vi "conditioning_behavior_120720.vi"() -> ()   [LabVIEW 2019]
doc: "The myRIO Project template acquires acceleration data from the onboard accelerometer and displays the changes of acceleration values in a waveform chart."
uses:
  <vilib>/myRIO/Common/Instrument Driver Framework/myRIO v1.0/Encoder/typedefs/Encoder Signal Mode.ctl
  <vilib>/myRIO/Instrument Drivers/Onboard IO/Encoder/typedefs/Encoder Reference.ctl
  <vilib>/myRIO/Common/Instrument Driver Framework/Utilities/typedefs/myRIO Generic Hardware Reference.ctl
  <vilib>/myRIO/Common/Instrument Driver Framework/Utilities/typedefs/Hardware Version Enum.ctl
  <vilib>/myRIO/Common/Instrument Driver Framework/Utilities/typedefs/myRIO v1.0 Reference.ctl
  <vilib>/myRIO/Common/Instrument Driver Framework/Utilities/typedefs/Generic FPGA Reference.ctl
  <vilib>/myRIO/Common/Instrument Driver Framework/myRIO v1.0/Encoder/typedefs/Encoder Channels Enum.ctl
  <vilib>/myRIO/Common/Instrument Driver Framework/myRIO v1.0/Encoder/typedefs/Encoder Configuration v1.0.ctl
  <vilib>/userdefined/High Color/nirio_resource_hc.ctl
  <vilib>/myRIO/Instrument Drivers/Onboard IO/DIO/typedefs/DIO Reference.ctl
  <vilib>/myRIO/Common/Instrument Driver Framework/myRIO v1.0/DIO/typedefs/DIO Channels List.ctl
  <vilib>/myRIO/Common/Instrument Driver Framework/myRIO v1.0/DIO/typedefs/DIO Channels Enum.ctl
  <vilib>/myRIO/Common/Instrument Driver Framework/Utilities/vis/Is FPGA Ref Available.vi
  <vilib>/myRIO/Common/Instrument Driver Framework/myRIO v1.0/Encoder/vis/myRIO v1.1 Open Encoder.vi
  <vilib>/myRIO/Instrument Drivers/Onboard IO/Encoder/vis/Read.vi
  <vilib>/myRIO/Common/Instrument Driver Framework/myRIO v1.0/DIO/vis/myRIO v1.1 Open DIO.vi
  <vilib>/myRIO/Instrument Drivers/Onboard IO/DIO/vis/Write.vi
  <vilib>/myRIO/Instrument Drivers/Onboard IO/DIO/vis/Read.vi
  <vilib>/myRIO/Common/Instrument Driver Framework/Utilities/vis/Validate Channels.vi
  <vilib>/myRIO/Common/Instrument Driver Framework/myRIO v1.0/Encoder/vis/myRIO v1.0 Reserve Encoder.vi
  <vilib>/myRIO/Common/Instrument Driver Framework/myRIO v1.0/DIO/vis/myRIO v1.0 Reserve DIO.vi
  <vilib>/myRIO/Common/Instrument Driver Framework/myRIO v1.0/Encoder/vis/myRIO v1.0 Build MUX Configuration Encoder.vi
  <vilib>/myRIO/Common/Instrument Driver Framework/myRIO v1.0/Resource Manager/vis/myRIO v1.0 Reserve Channel List.vi
  <vilib>/myRIO/Common/Instrument Driver Framework/myRIO v1.0/DIO/vis/myRIO v1.0 Build MUX Configuration DIO.vi
  <vilib>/myRIO/Common/Instrument Driver Framework/myRIO v1.0/Resource Manager/vis/myRIO v1.0 Create Configuration List.vi
  <vilib>/myRIO/Common/Instrument Driver Framework/myRIO v1.0/Resource Manager/vis/myRIO v1.0 Reserve Channel.vi
  <vilib>/myRIO/Common/Instrument Driver Framework/myRIO v1.0/Resource Manager/vis/myRIO v1.0 Unreserve Channel.vi
  <vilib>/myRIO/Common/Instrument Driver Framework/myRIO v1.0/Resource Manager/vis/myRIO v1.0 Build Mutex Name.vi
  <vilib>/Utility/VariantDataType/GetNumericInfo.vi
  <vilib>/Utility/error.llb/Error Cluster From Error Code.vi
  <vilib>/myRIO/Common/Instrument Driver Framework/myRIO v1.0/myRIO v1.1 Open.vi
  <vilib>/myRIO/Common/Instrument Driver Framework/Utilities/vis/IO Manager.vi
  <vilib>/myRIO/Common/Instrument Driver Framework/Utilities/vis/Configuration Manager.vi
  <vilib>/myRIO/Common/Instrument Driver Framework/myRIO v1.0/Resource Manager/vis/myRIO v1.0 Configure IO.vi
  <vilib>/myRIO/Common/Instrument Driver Framework/myRIO v1.0/myRIO v1.0 Close.vi
  <vilib>/myRIO/Common/Instrument Driver Framework/myRIO v1.0/Encoder/vis/myRIO v1.0 Configure Encoder.vi
  <vilib>/myRIO/Common/Instrument Driver Framework/myRIO v1.0/Encoder/vis/myRIO v1.0 Read Encoder.vi
  <vilib>/myRIO/Common/Instrument Driver Framework/myRIO v1.0/DIO/vis/myRIO v1.0 Read DIO.vi
  <vilib>/myRIO/Common/Instrument Driver Framework/myRIO v1.0/DIO/vis/myRIO v1.0 Write DIO.vi
  <vilib>/myRIO/Express VI/Onboard IO/Encoder/Encoder Express VI.xnode
  <vilib>/myRIO/Instrument Drivers/Onboard IO/Encoder/vis/myRIO Encoder Open.xnode
  <vilib>/myRIO/Express VI/Onboard IO/DI/DI Express VI.xnode
  <vilib>/myRIO/Instrument Drivers/Onboard IO/DIO/vis/myRIO DIO Open.xnode
  <vilib>/myRIO/Express VI/Onboard IO/DO/DO Express VI.xnode
  <vilib>/myRIO/Instrument Drivers/Onboard IO/Encoder/Encoder.lvlib
  <vilib>/myRIO/Instrument Drivers/Onboard IO/DIO/DIO.lvlib
panel:
  out "Frame clock":i32
  out "Reward":bool=TRUE
  in  "Give reward":bool
  out "Licks":u32
  out "Lick":bool
  out "Output":dbl[][](array[numeric])
  out "Time":dbl
  out "Display":bool
  out "Stop":bool
  in  "Frames to collect":u32
  out "Overflow?":bool
  out "Counter Value":i32
  out "Velocity":dbl
  out "Velocity Plot":dbl[](graph)
  out "Velocity array":dbl[](array[numeric])
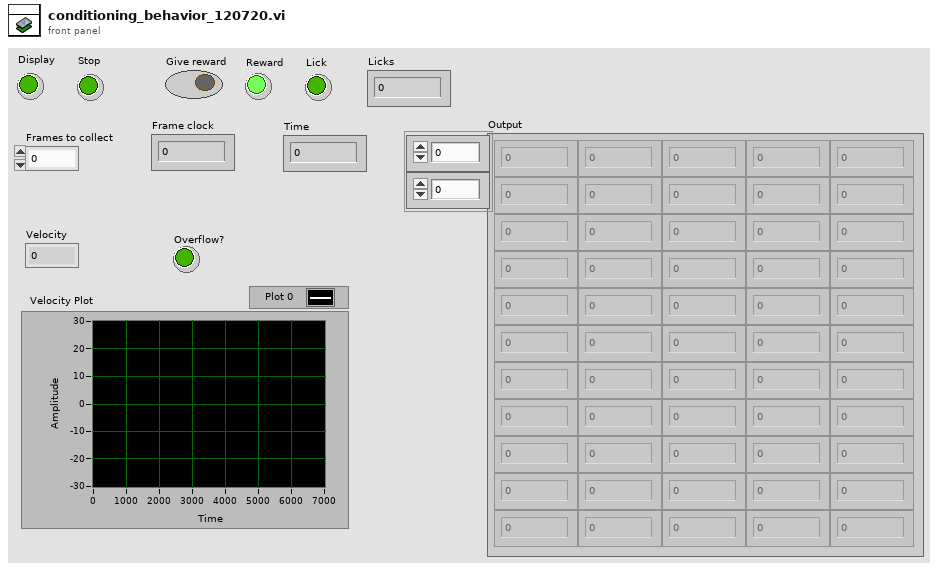
[diagram p1: front panel]
types:
  T1 = typedef "Encoder.lvlib/Encoder Reference.ctl" = cluster{"myRIO Reference":T2, "Encoder Channels Enum":T6}
  T2 = typedef "myRIO Generic Hardware Reference.ctl" = cluster{"myRIO Model":T3, "myRIO Hardware Reference":T4}
  T3 = typedef "Hardware Version Enum.ctl" = enum16{"Unknown", "myRIO-1900", "myRIO-1950", "roboRIO", "NI ELVIS RIO CM", "ELVIS III"}
  T4 = typedef "myRIO v1.0 Reference.ctl" = cluster{"Generic FPGA Reference":T5, "Allow multiple opens":bool}
  T5 = typedef "Generic FPGA Reference.ctl" = refnum<k20>
  T6 = typedef "Encoder Channels Enum.ctl" = enum16{"Not Connected", "C/ENC0", "C/ENC1", "A/ENC", "A/ENC0", "A/ENC1", "A/ENC2", "A/ENC3", "A/ENC4", "A/ENC5", "A/ENC6", "A/ENC7", "A/ENC8", "A/ENC9", "B/ENC", "B/ENC0", "B/ENC1", "B/ENC2", "B/ENC3", "B/ENC4", "B/ENC5", "B/ENC6", "B/ENC7", "B/ENC8", "B/ENC9", "DIO/ENC0", "DIO/ENC1", "DIO/ENC2", "DIO/ENC3", "DIO/ENC4"}
  T7 = typedef "Encoder Signal Mode.ctl" = enum16{"Quadrature phase signal", "Step and direction signal"}
  T8 = typedef "nirio_resource_hc.ctl" = tag
  T9 = typedef "DIO.lvlib/DIO Reference.ctl" = cluster{"myRIO Reference":T2, "DIO Channels List":T10}
  T10 = typedef "DIO Channels List.ctl" = T11[]
  T11 = typedef "DIO Channels Enum.ctl" = enum16{"Not Connected", "C/DIO0", "C/DIO1", "C/DIO2", "C/DIO3", "C/DIO4", "C/DIO5", "C/DIO6", "C/DIO7", "A/DIO0", "A/DIO1", "A/DIO2", "A/DIO3", "A/DIO4", "A/DIO5", "A/DIO6", "A/DIO7", "A/DIO8", "A/DIO9", "A/DIO10", "A/DIO11", "A/DIO12", "A/DIO13", "A/DIO14", "A/DIO15", "A/DIO16", "A/DIO17", "A/DIO18", "A/DIO19", "B/DIO0", "B/DIO1", "B/DIO2", "B/DIO3", "B/DIO4", "B/DIO5", "B/DIO6", "B/DIO7", "B/DIO8", "B/DIO9", "B/DIO10", "B/DIO11", "B/DIO12", "B/DIO13", "B/DIO14", "B/DIO15", "B/DIO16", "B/DIO17", "B/DIO18", "B/DIO19", "LED0", "LED1", "LED2", "LED3", "Button0", "DIO/DIO0", "DIO/DIO1", "DIO/DIO2", "DIO/DIO3", "DIO/DIO4", "DIO/DIO5", "DIO/DIO6", "DIO/DIO7", "DIO/DIO8", "DIO/DIO9", "SPI/CS0", "SPI/CS1", "SPI/CS2", "SPI/CS3", "LED RADIO (Green)", "LED RADIO (Red)", "LED COMM (Green)", "LED COMM (Red)", "LED MODE (Green)", "LED MODE (Red)"}
  T12 = typedef "NI_Matrix.lvlib/RealMatrix.ctl" = dbl[][]
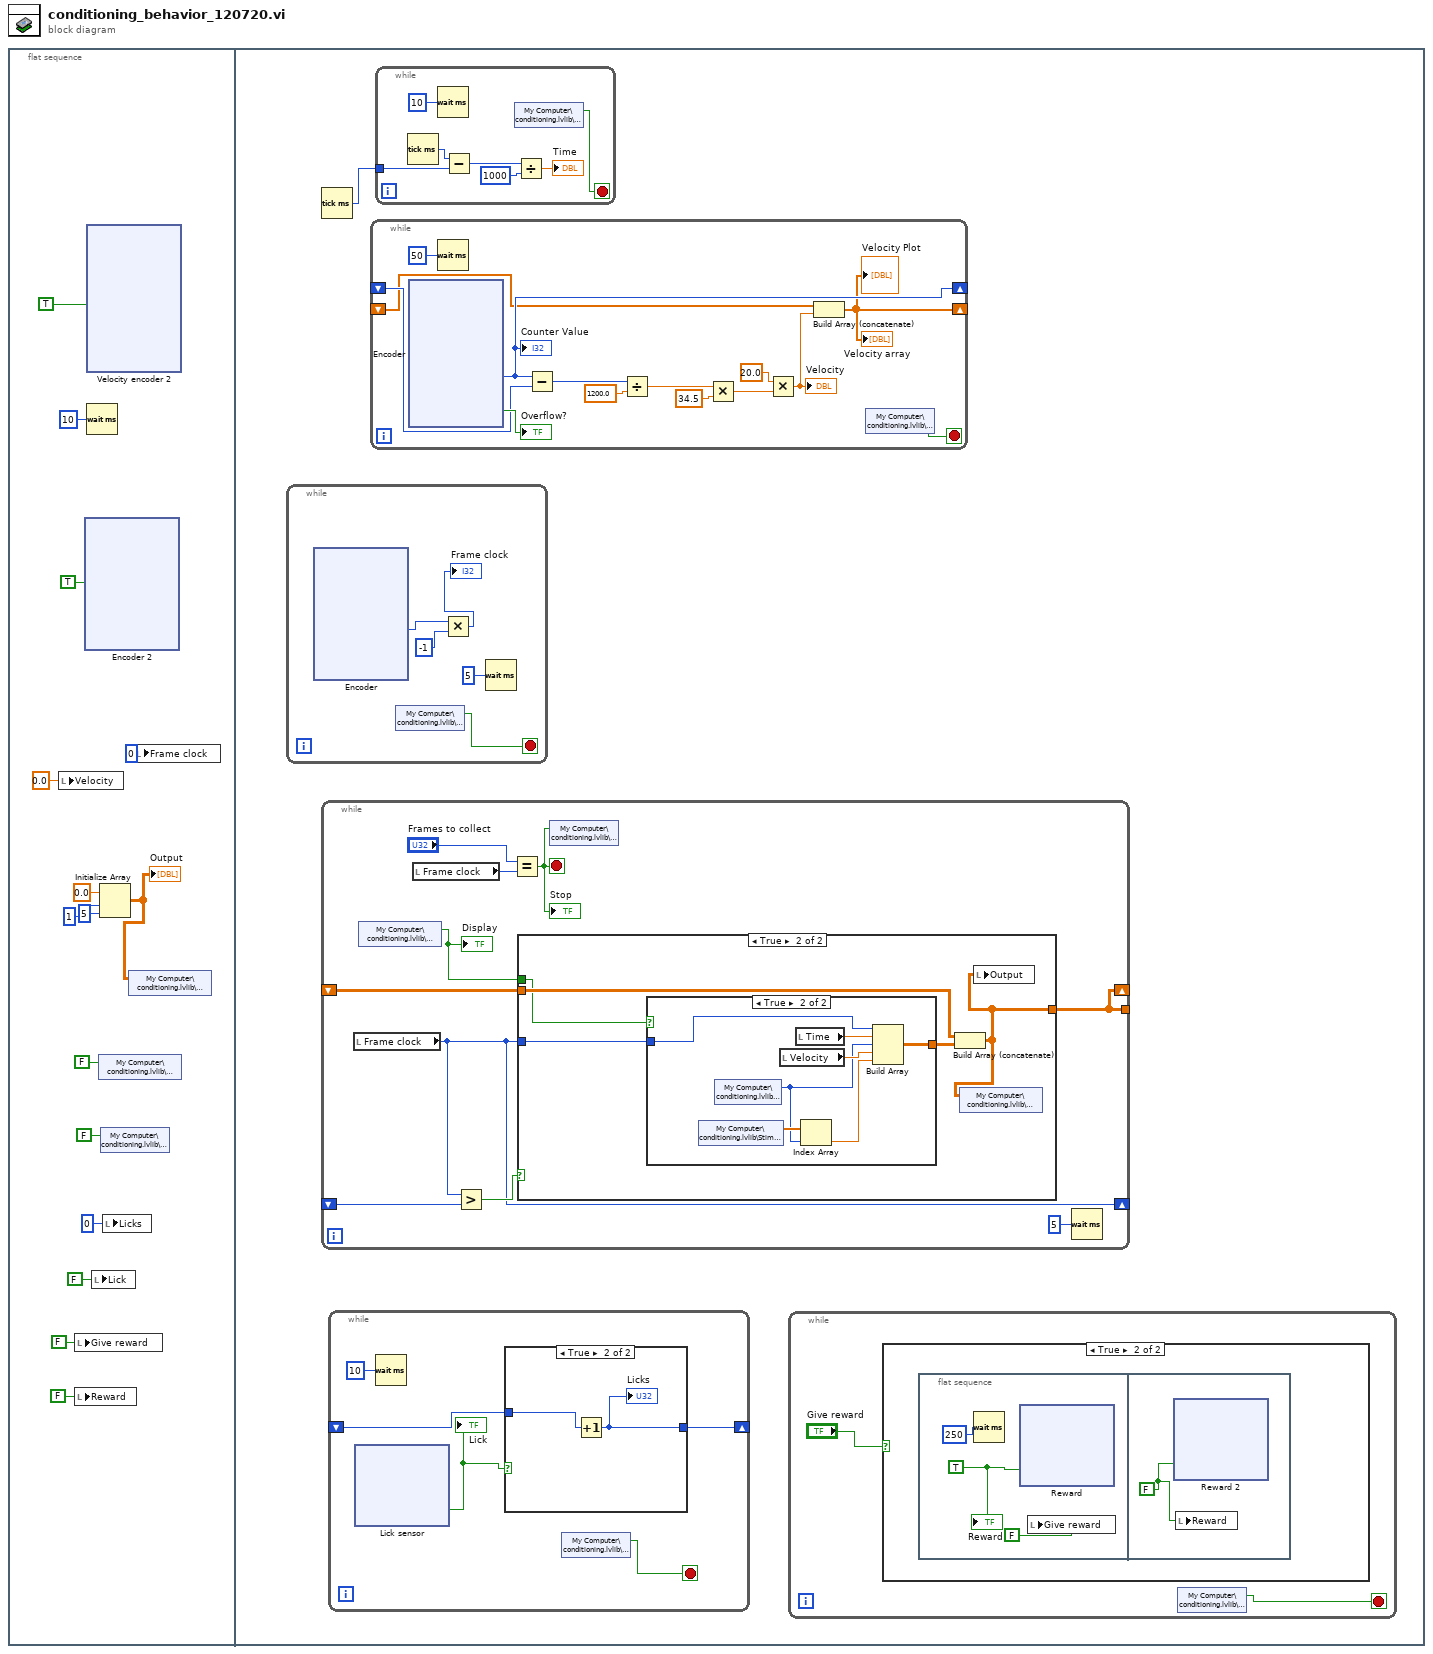
[diagram p0: block diagram]
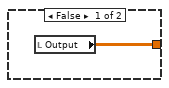
[diagram p4: hidden frame]
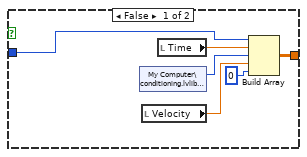
[diagram p5: hidden frame]
diagram:
  n1 = flat-sequence {
    frame #0 {
      n2 = local write "Velocity"(0.0 ("Velocity")) -> ()
      n3 = local write "Give reward"(FALSE ("Give reward")) -> ()
      n4 = local write "Reward"(FALSE ("Reward")) -> ()
      n5 = xnode "Encoder 2"("Reset Counter"=TRUE) -> ()  [unwired: 1 in, 4 out]
      n6 = xnode "Velocity encoder 2"("Reset Counter"=TRUE) -> ()  [unwired: 1 in, 4 out]
      n7 = Wait (ms)(milliseconds to wait=u32 10) -> ()  [unwired: 1 out]
      n8 = local write "Lick"(FALSE ("Lick")) -> ()
      n9 = shared-variable "My Computer\\conditioning.lvlib\\Display"(FALSE ("Display")) -> ()  [unwired: 1 in, 1 out]
      n10 = Initialize Array(0.0 ("element"), 1 ("dimension size"), 5 ("dimension size")) -> (w9:dbl[][])
      "Output" <- w9
      n11 = shared-variable "My Computer\\conditioning.lvlib\\Stop"(FALSE ("Stop")) -> ()  [unwired: 1 in, 1 out]
      n12 = local write "Licks"(u32 0 ("Licks")) -> ()
      n13 = shared-variable "My Computer\\conditioning.lvlib\\Output"(w9) -> ()  [unwired: 1 in, 1 out]
      n14 = local write "Frame clock"(u32 0 ("Frames")) -> ()
    }
    frame #1 {
      n15 = while {
        stop <- w110 stop-if-true
        n16 = xnode "Encoder"() -> ("Counter Value"=w113:i32)  [unwired: 2 in, 3 out]
        n17 = shared-variable "My Computer\\conditioning.lvlib\\Stop"() -> (w110:bool)  [unwired: 1 in, 1 out]
        n18 = Multiply(x=w113, y=-1) -> (x*y=→"Frame clock":i32)
        n19 = Wait (ms)(milliseconds to wait=u32 5) -> ()  [unwired: 1 out]
      }
      n20 = Tick Count (ms)() -> (millisecond timer value=w108:u32)
      n21 = while {
        shift-right: [w353] -> _
        shift-left: _ -> [w355]
        shift-right: [w348] -> _
        shift-left: _ -> [w352]
        tunnel: [w348] -> _
        stop <- w347 stop-if-true
        n22 = local read "Frame clock"() -> (w353:i32)
        n23 = shared-variable "My Computer\\conditioning.lvlib\\Display"() -> (w346:bool)  [unwired: 1 in, 1 out]
        "Display" <- w346
        n24 = local read "Frame clock"() -> (w350:i32)
        n25 = Greater?(x=w353, y=w355) -> (0:w354:bool)
        n26 = Equal?(x="Frames to collect", y=w350) -> (x = y?=w347:bool)
        "Stop" <- w347
        n27 = case shown="True" w354 {
          tunnel: w353 -> [_ w361]
          tunnel: w352 -> [_ w360]
          tunnel: [w356 w357] -> w348
          tunnel: w346 -> [_ w358]
          frame False {
            n28 = local read "Output"() -> (w356:dbl[][])
          }
          frame True {
            n29 = case shown="True" w358 {
              tunnel: w361 -> [w362 w374]
              tunnel: [w366 w373] -> w359
              frame False {
                n30 = shared-variable "My Computer\\conditioning.lvlib\\Trial"() -> (w364:u32)  [unwired: 1 in, 1 out]
                n31 = local read "Velocity"() -> (w363:dbl)
                n32 = local read "Time"() -> (w365:dbl)
                n33 = Build Array(w362, w365, w364, w363, 0) -> (w366:T12)
              }
              frame True {
                n34 = shared-variable "My Computer\\conditioning.lvlib\\Stim_ID"() -> (w370:dbl[])  [unwired: 1 in, 1 out]
                n35 = shared-variable "My Computer\\conditioning.lvlib\\Trial"() -> (w369:u32)  [unwired: 1 in, 1 out]
                n36 = local read "Velocity"() -> (w371:dbl)
                n37 = local read "Time"() -> (w372:dbl)
                n38 = Index Array(array=w370, index=w369) -> (element=w368:dbl)
                n39 = Build Array(w374, w372, w369, w371, w368) -> (w373:T12)
              }
            }
            n40 = Build Array (concatenate)(w360, w359) -> (w357:T12)
            n41 = shared-variable "My Computer\\conditioning.lvlib\\Output"(w357) -> ()  [unwired: 1 in, 1 out]
            n42 = local write "Output"(w357) -> ()
          }
        }
        n43 = shared-variable "My Computer\\conditioning.lvlib\\Stop"(w347) -> ()  [unwired: 1 in, 1 out]
        n44 = Wait (ms)(milliseconds to wait=u32 5) -> ()  [unwired: 1 out]
      }
      n45 = while {
        shift-right: [w237] -> _
        shift-left: _ -> [w236]
        stop <- w240 stop-if-true
        n46 = xnode "Lick sensor"() -> ("C/DIO1 (DIO1)"=w238:bool)  [unwired: 1 in, 1 out]
        "Lick" <- w238
        n47 = Wait (ms)(milliseconds to wait=u32 10) -> ()  [unwired: 1 out]
        n48 = case shown="True" w238 {
          tunnel: [w241 w243] -> w237
          tunnel: w236 -> [w241 w242]
          frame False {
          }
          frame True {
            n49 = Increment(x=w242) -> (x+1=w243:u32)
            "Licks" <- w243
          }
        }
        n50 = shared-variable "My Computer\\conditioning.lvlib\\Stop"() -> (w240:bool)  [unwired: 1 in, 1 out]
      }
      n51 = while {
        shift-right: [w289] -> _
        shift-left: _ -> [w290]
        shift-right: [w281] -> _
        shift-left: _ -> [w280]
        stop <- w279 stop-if-true
        n52 = xnode "Encoder"() -> ("Counter Value"=w289:i32, "Overflow?"=→"Overflow?":bool)  [unwired: 2 in, 2 out]
        "Counter Value" <- w289
        n53 = Wait (ms)(milliseconds to wait=u32 50) -> ()  [unwired: 1 out]
        n54 = Subtract(x=w289, y=w290) -> (x-y=w282:i32)
        n55 = Divide(x=w282, y=1200.0 ("600")) -> (x/y=w287:dbl)
        n56 = Multiply(x=w287, y=34.5) -> (x*y=w285:dbl)
        n57 = Multiply(x=20.0, y=w285) -> (x*y=w283:dbl)
        "Velocity" <- w283
        n58 = Build Array (concatenate)(w280, w283) -> (w281:dbl[])
        "Velocity Plot" <- w281
        "Velocity array" <- w281
        n59 = shared-variable "My Computer\\conditioning.lvlib\\Stop"() -> (w279:bool)  [unwired: 1 in, 1 out]
      }
      n60 = while {
        tunnel: w108 -> [w344]
        stop <- w339 stop-if-true
        n61 = Tick Count (ms)() -> (millisecond timer value=w345:u32)
        n62 = Wait (ms)(milliseconds to wait=u32 10) -> ()  [unwired: 1 out]
        n63 = Subtract(x=w345, y=w344) -> (x-y=w342:u32)
        n64 = shared-variable "My Computer\\conditioning.lvlib\\Stop"() -> (w339:bool)  [unwired: 1 in, 1 out]
        n65 = Divide(x=w342, y=u32 1000) -> (x/y=→"Time":dbl)
      }
      n66 = while {
        stop <- w160 stop-if-true
        n67 = case shown="True" "Give reward" {
          frame False {
          }
          frame True {
            n68 = flat-sequence {
              frame #0 {
                w164 = TRUE ("C/DIO0 (DIO0)")
                n69 = Wait (ms)(milliseconds to wait=u32 250) -> ()  [unwired: 1 out]
                n70 = xnode "Reward"("C/DIO0 (DIO0)"=w164) -> ()  [unwired: 1 in, 1 out]
                n71 = local write "Give reward"(FALSE ("Give reward")) -> ()
                "Reward" <- w164
              }
              frame #1 {
                w200 = FALSE ("C/DIO0 (DIO0)")
                n72 = xnode "Reward 2"("C/DIO0 (DIO0)"=w200) -> ()  [unwired: 1 in, 1 out]
                n73 = local write "Reward"(w200) -> ()
              }
            }
          }
        }
        n74 = shared-variable "My Computer\\conditioning.lvlib\\Stop"() -> (w160:bool)  [unwired: 1 in, 1 out]
      }
    }
  }
